vi "ASK_DeSync.vi"(8 "error in (no error)":errorcluster caption="错误输入（无错误）", 10 "judge_data":dbl[](array[numeric]) format="%#_13g", 11 "PathIn":path) -> (0 "error out":errorcluster caption="错误输出", 2 "data1":dbl[](array[numeric]), 3 "PathOut":path)   [LabVIEW 2015]
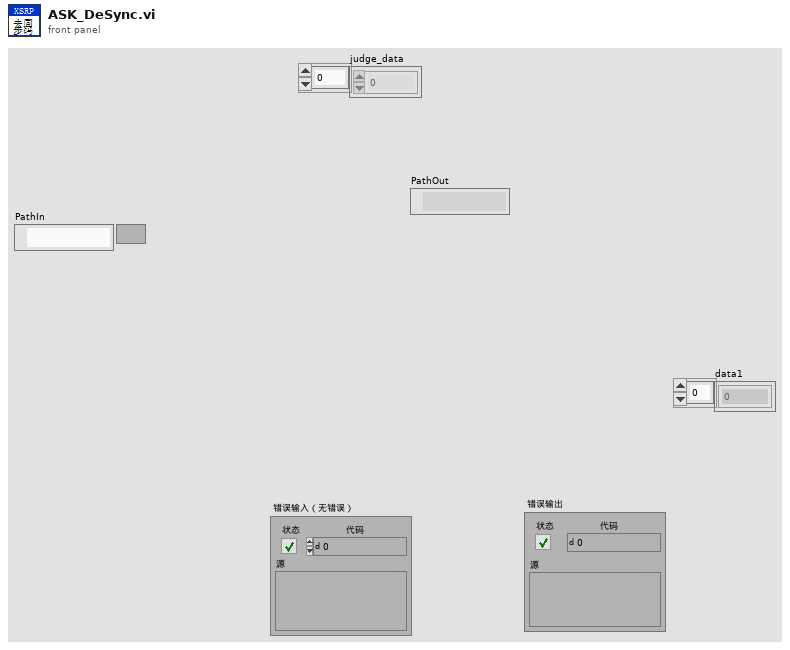
[diagram p1: front panel]
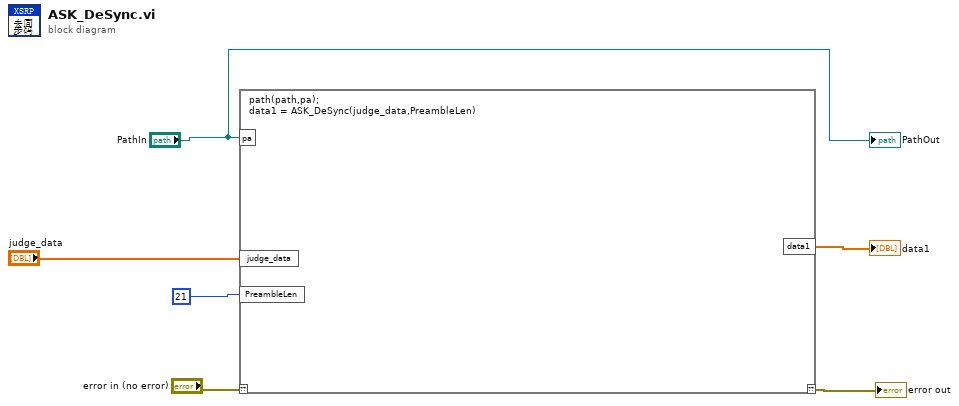
[diagram p0: block diagram]
diagram:
  n1 = script code="path(path,pa);\ndata1 = ASK_DeSync(judge_data,PreambleLen)"("??"="error in (no error)", "pa"="PathIn", "judge_data"="judge_data", "PreambleLen"=21) -> ("??"=→"error out":errorcluster, "data1"=→"data1":dbl[])
  "PathOut" <- "PathIn"
